vi "try_to_calibrate.vi"() -> ()   [LabVIEW 2014]
uses:
  <vilib>/Utility/file.llb/Read From Spreadsheet File (DBL).vi
panel:
  out "transposed array":dbl[][](array[numeric])
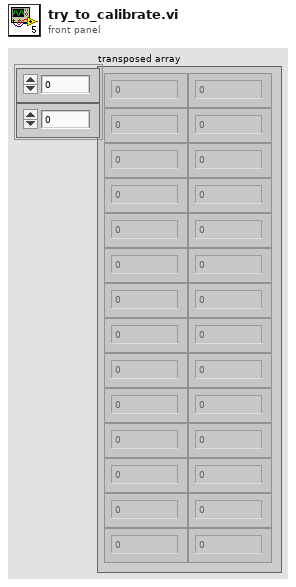
[diagram p1: front panel]
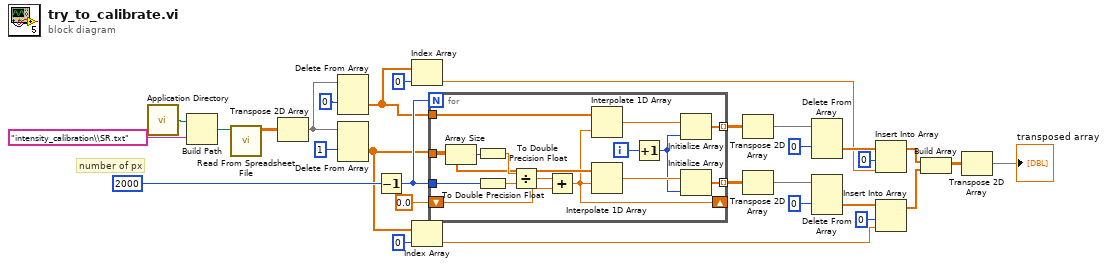
[diagram p0: block diagram]
diagram:
  # "number of px"
  n1 = call <vilib>:"Application Directory.vi"() -> ("Application Directory"=w30:path)
  n2 = Build Path(base path=w30, name or relative path="intensity_calibration\\SR.txt") -> (appended path=w29:path)
  n3 = call-poly <vilib>:"Read From Spreadsheet File.vi"("file path (dialog if empty)"=w29) -> ("all rows"=w26:dbl[][])  [unwired: 6 in, 4 out]
  n4 = Transpose 2D Array(2D array=w26) -> (transposed array=w17:dbl[][])
  n5 = Delete From Array(array=w17, index (row)=0 ("length")) -> (deleted portion=w12:dbl[])  [unwired: 2 in, 1 out]
  n6 = Delete From Array(array=w17, index (row)=1) -> (deleted portion=w9:dbl[])  [unwired: 2 in, 1 out]
  n7 = Decrement(x=2000) -> (x-1=w22:i32)
  n8 = Index Array(array=w12, index=0) -> (element=w7:dbl)
  n9 = Index Array(array=w9, index=0) -> (element=w2:dbl)
  n10 = for {
    N: w22 -> [_]
    tunnel: w9 -> [w34]
    tunnel: w22 -> [w37]
    tunnel: [w43] -> w24 mode=indexing
    shift-right: [w32] -> _
    shift-left: 0.0 -> [w41]
    tunnel: [w35] -> w15 mode=indexing
    tunnel: w12 -> [w33]
    i -> [w44]
    n11 = Array Size(array=w34) -> (size(s)=w39:i32)
    n12 = To Double Precision Float(number=w39) -> (double precision float=w40:dbl)
    n13 = To Double Precision Float(number=w37) -> (double precision float=w38:dbl)
    n14 = Divide(x=w40, y=w38) -> (x/y=w42:dbl)
    n15 = Add(x=w42, y=w41) -> (x+y=w32:dbl)
    n16 = Interpolate 1D Array(1:w32, 2:w33) -> (0:w31:dbl)
    n17 = Interpolate 1D Array(1:w32, 2:w34) -> (0:w45:dbl)
    n18 = Increment(x=w44) -> (x+1=w36:i32)
    n19 = Initialize Array(w31, w36) -> (w35:dbl[])
    n20 = Initialize Array(w45, w36) -> (w43:dbl[])
  }
  n21 = Transpose 2D Array(2D array=w15) -> (transposed array=w14:dbl[][])
  n22 = Transpose 2D Array(2D array=w24) -> (transposed array=w20:dbl[][])
  n23 = Delete From Array(array=w14, index (row)=0) -> (deleted portion=w8:dbl[])  [unwired: 2 in, 1 out]
  n24 = Delete From Array(array=w20, index (row)=0) -> (deleted portion=w3:dbl[])  [unwired: 2 in, 1 out]
  n25 = Insert Into Array(array=w8, index=0, new element=w7) -> (w5:dbl[])
  n26 = Insert Into Array(array=w3, index=0, new element=w2) -> (w1:dbl[])
  n27 = Build Array(w5, w1) -> (w18:dbl[][])
  n28 = Transpose 2D Array(2D array=w18) -> (transposed array=→"transposed array":dbl[][])
